vi "Select.vi"(10 "Line":u8, 11 "Text.Text":string) -> (1 "scale":i32, 2 "Text min":i32, 3 "Text max":i32)   [LabVIEW 2016]
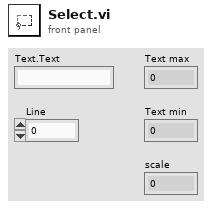
[diagram p1: front panel]
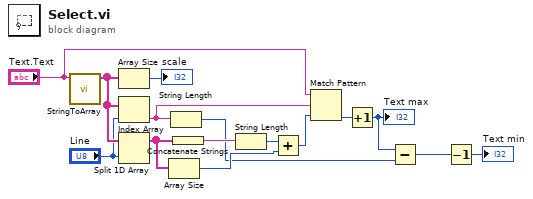
[diagram p0: block diagram]
diagram:
  n1 = call "StringToArray.vi"("write buffer"="Text.Text") -> ("Array"=w12:string[])  [unwired: 10 in]
  n2 = Array Size(array=w12) -> (size(s)=→"scale":i32)
  n3 = Index Array(array=w12, index="Line") -> (element=w7:string)
  n4 = Split 1D Array(array=w12, index="Line") -> (first subarray=w9:string[])  [unwired: 1 out]
  n5 = Array Size(array=w9) -> (size(s)=w10:i32)
  n6 = String Length(string=w7) -> (length=w2:i32)
  n7 = Concatenate Strings(w9) -> (w5:string)
  n8 = String Length(string=w5) -> (length=w8:i32)
  n9 = Add(x=w8, y=w10) -> (x+y=w11:i32)
  n10 = Match Pattern(string="Text.Text", regular expression=w7, offset (0)=w11) -> (offset past match=w3:i32)  [unwired: 3 out]
  n11 = Increment(x=w3) -> (x+1=w14:i32)
  "Text max" <- w14
  n12 = Subtract(x=w14, y=w2) -> (x-y=w4:i32)
  n13 = Decrement(x=w4) -> (x-1=→"Text min":i32)
